vi "Complementary Incomplete Gamma Function.vi"(2 "a":dbl=inf format="%.2f", 3 "x":dbl format="%.2f") -> (1 "1 - g(x, a)":dbl format="%.2f")   [LabVIEW 2018, in "NI_Gmath.lvlib"]
doc: "Computes the complementary incomplete gamma function."
uses:
  NI_Gmath.lvlib
  <resource>/lvanlys.dll
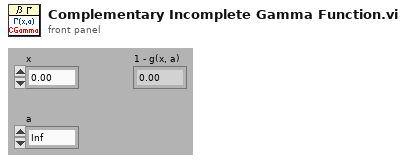
[diagram p1: front panel]
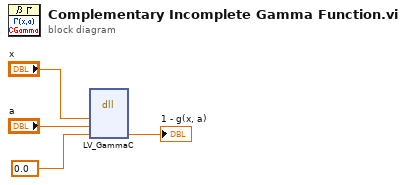
[diagram p0: block diagram]
diagram:
  n1 = dll-call lib="C:/Program Files (x86)/National Instruments/LabVIEW 2018/resource/lvanlys.*" fn="LV_GammaC"("x"="x", "a"="a", "GammaC(x, a)"=0.0 ("GammaC")) -> ("GammaC(x, a)"=→"1 - g(x, a)":dbl)  [unwired: 6 in, 2 out]
